vi "FPGAReadout.vi"() -> ()   [LabVIEW 2018]
uses:
  Downloads/hx711 myRIO/hx711/State.ctl
  Downloads/hx711 myRIO/hx711/Data.ctl
  <vilib>/rvi/Emulation/niFpgaGetClockAttributes.vi
  <vilib>/rvi/Emulation/niFpgaSctlEmulationGetInTimedLoop.vi
  <vilib>/rvi/Emulation/niFpgaEmulationReportErrorSimple.vi
  <vilib>/rvi/Emulation/niFpgaProcessEmulError.vi
  <vilib>/rvi/eio/common/nirviEmuTemplateMethod_errors.vi
  <vilib>/rvi/Emulation/niFpgaCriticalErrorInLSC.vi
  <vilib>/eio/EIONode/EIONode.xnode
panel:
  in  "PowerDown? 3":bool
  out "Data 3":i32
  in  "Gain/ChannelSelect 3":T1(ring)
  out "ConnectorA/DIO4":bool
  out "State 3":T2
  out "Data array3":i32[](array[numeric])
  in  "PowerDown? 2":bool
  out "Data 2":i32
  in  "Gain/ChannelSelect 2":T1(ring)
  out "ConnectorA/DIO2":bool
  out "State 2":T2
  out "Data array 2":i32[](array[numeric])
  out "RawCurrent":u16
  out "RawVoltage":i16
  out "State":T2
  out "ConnectorA/DIO0":bool
  out "Data array":i32[](array[numeric])
  in  "PowerDown?":bool
  out "Data":i32
  in  "Gain/ChannelSelect":T1(ring)
  in  "stop":bool
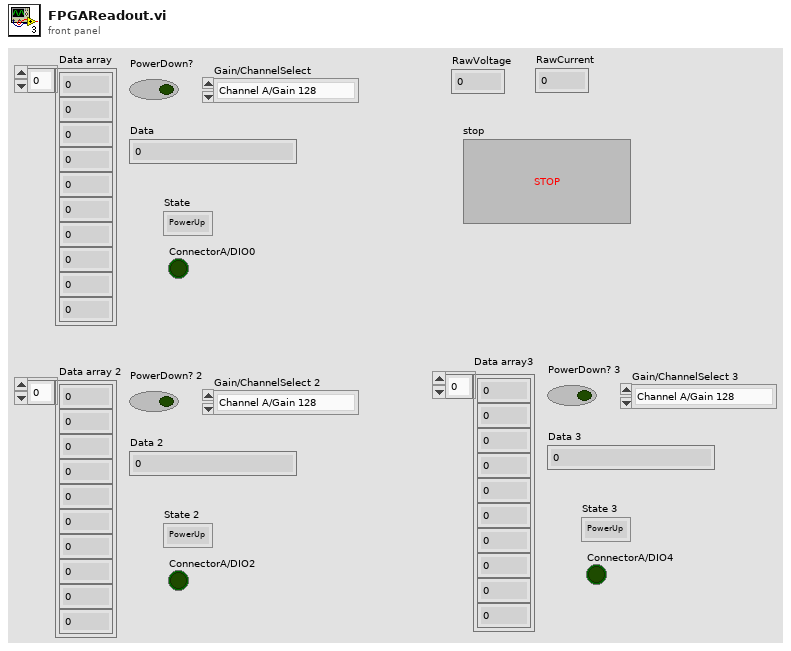
[diagram p1: front panel]
types:
  T1 = enum16{"Channel A/Gain 128", "Channel A/Gain 64", "Channel B/Gain 32"}
  T2 = typedef "State.ctl" = enum16{"PowerUp", "PowerDown", "Gain/ChannelSelect", "ReadData", "ClockLow", "ClockHigh", "ConvertData", "RetrievalReady?"}
  T3 = typedef "Data.ctl" = cluster{"DT":bool, "SCK":bool, "2's Data":i32, "PulseCount":u8, "DelayTime":u8, "Data":i32, "PowerDown?":bool, "Gain/ChannelSelect":enum16{"Channel A/Gain 128", "Channel A/Gain 64", "Channel B/Gain 32"}}
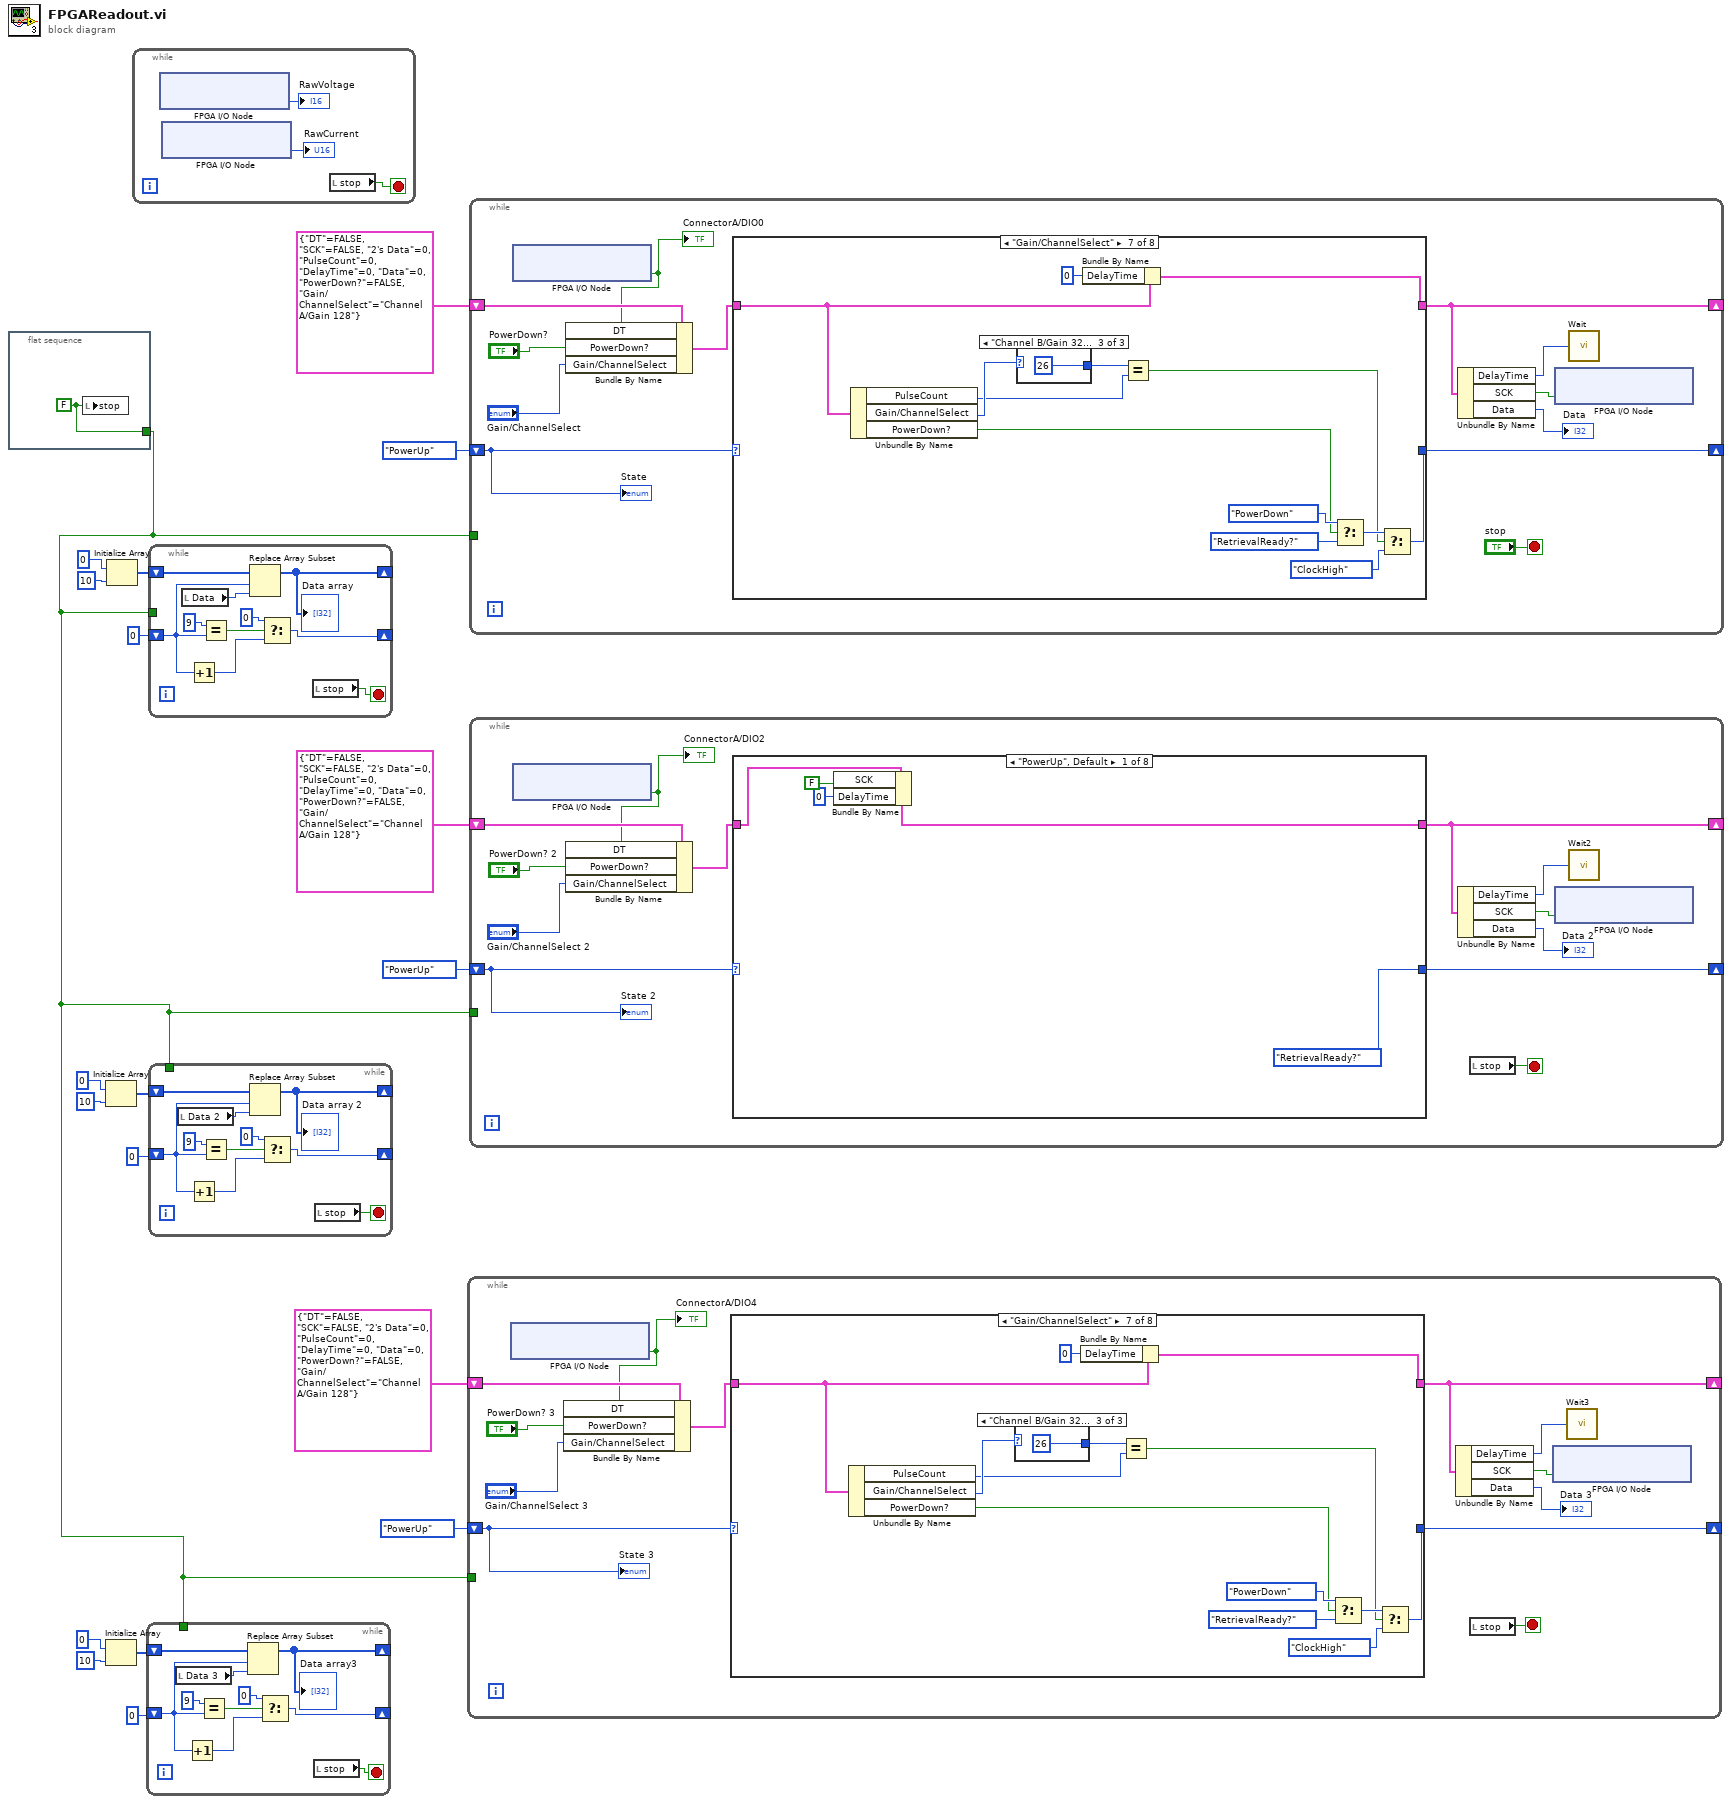
[diagram p0: block diagram]
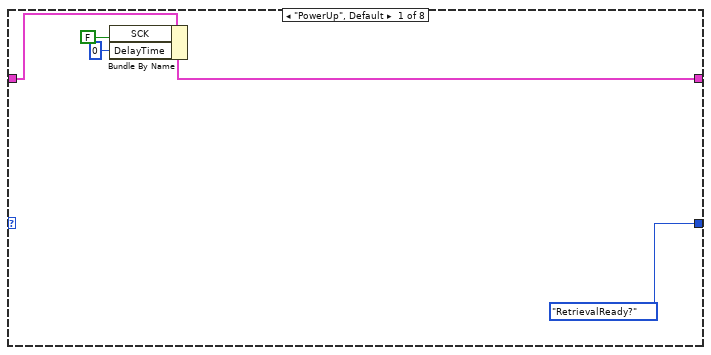
[diagram p2: hidden frame]
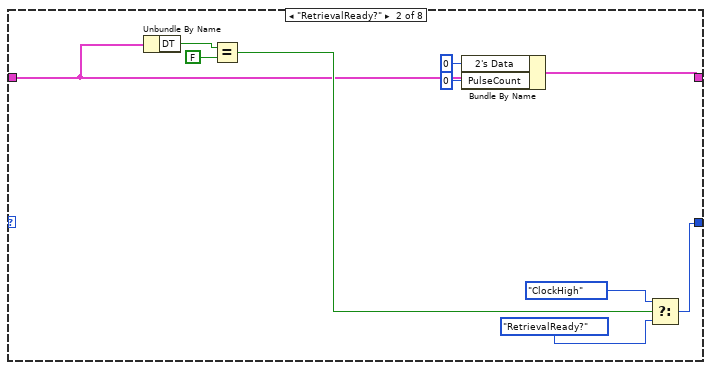
[diagram p3: hidden frame]
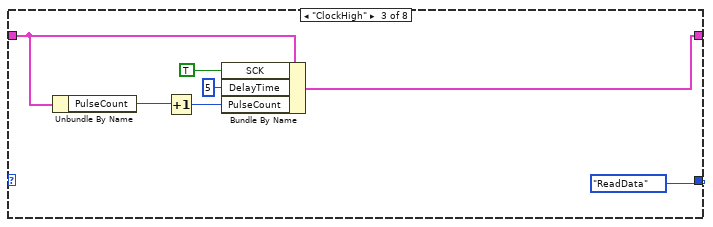
[diagram p4: hidden frame]
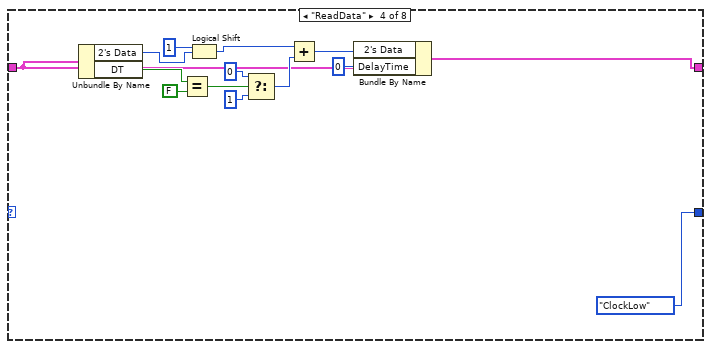
[diagram p5: hidden frame]
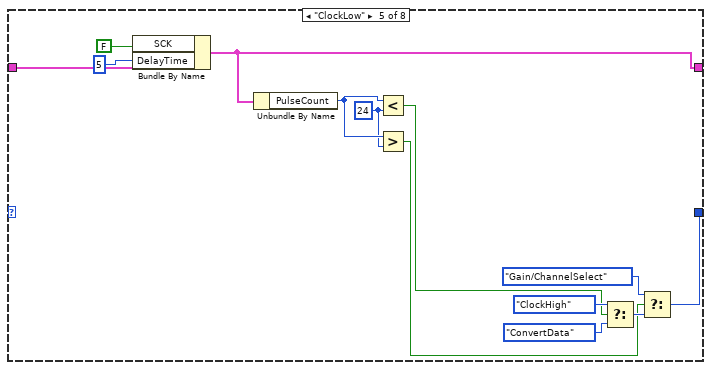
[diagram p6: hidden frame]
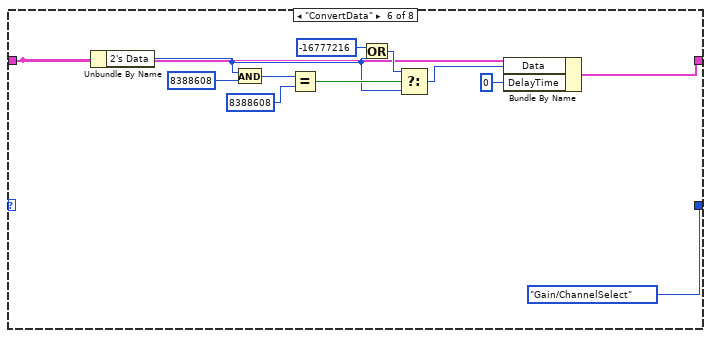
[diagram p7: hidden frame]
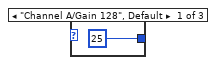
[diagram p8: hidden frame]
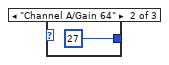
[diagram p9: hidden frame]
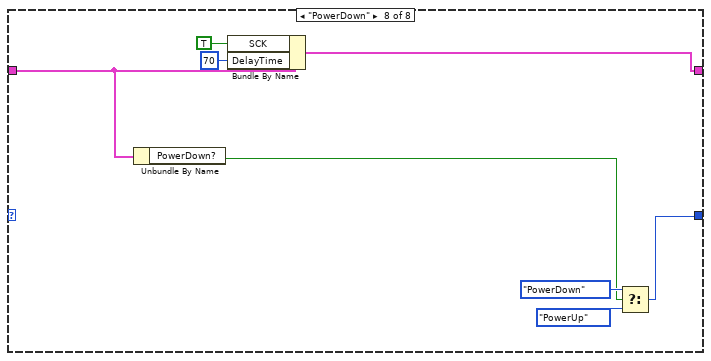
[diagram p10: hidden frame]
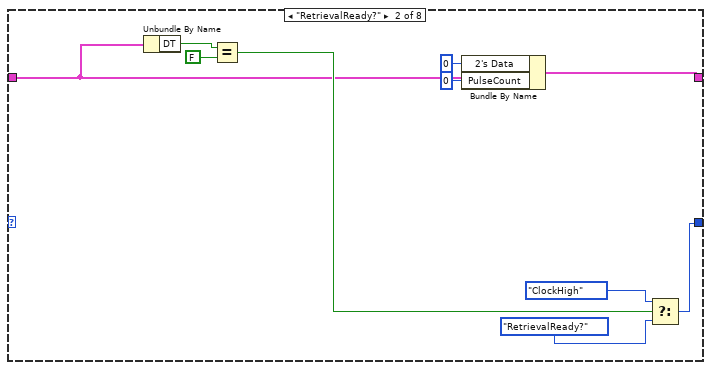
[diagram p11: hidden frame]
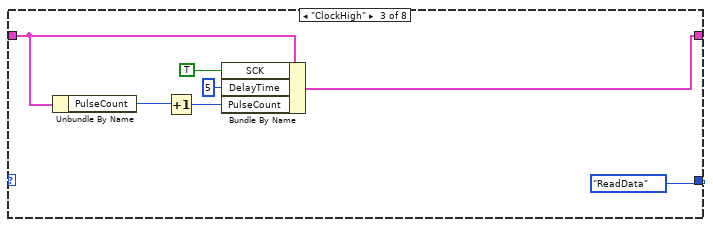
[diagram p12: hidden frame]
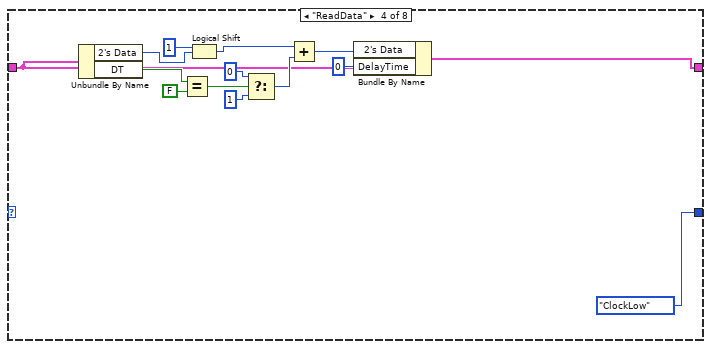
[diagram p13: hidden frame]
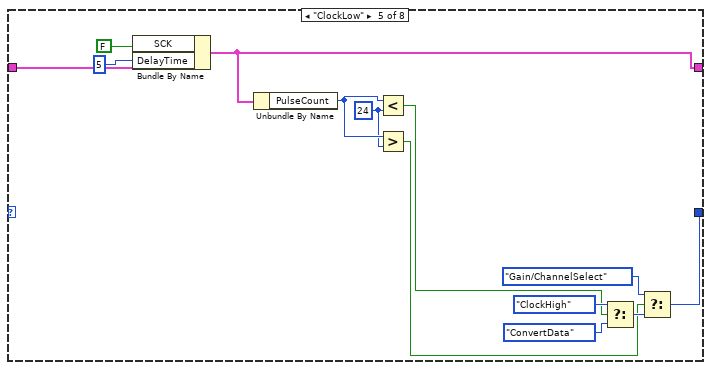
[diagram p14: hidden frame]
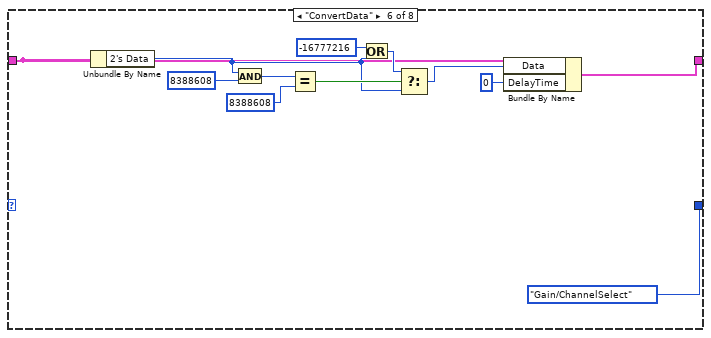
[diagram p15: hidden frame]
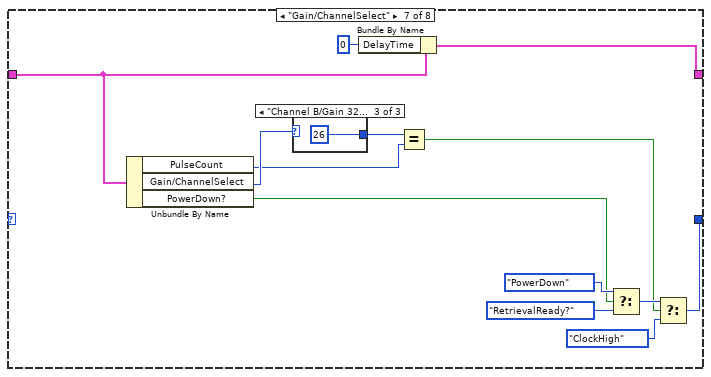
[diagram p16: hidden frame]
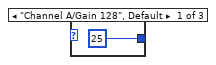
[diagram p17: hidden frame]
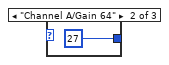
[diagram p18: hidden frame]
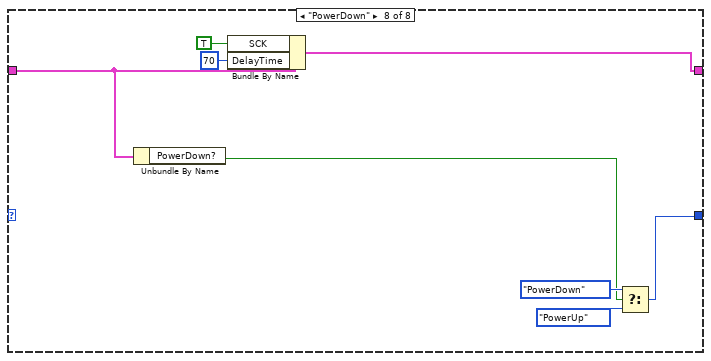
[diagram p19: hidden frame]
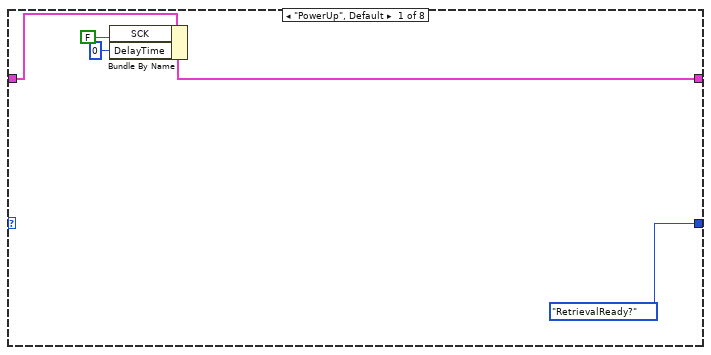
[diagram p20: hidden frame]
diagram:
  n1 = flat-sequence {
    tunnel: [w20] -> w9
    frame #0 {
      w20 = FALSE
      n2 = local write "stop"(w20) -> ()
    }
  }
  n3 = Initialize Array(0 ("Data"), 10 ("dimension size")) -> (w5:i32[])
  n4 = Initialize Array(0 ("Data"), 10 ("dimension size")) -> (w2:i32[])
  n5 = Initialize Array(0 ("Data"), 10 ("dimension size")) -> (w16:i32[])
  n6 = while {
    stop <- w21 stop-if-true
    n7 = xnode "FPGA I/O Node"() -> ("ConnectorC/AI0"=→"RawVoltage":i16)  [unwired: 1 in, 1 out]
    n8 = xnode "FPGA I/O Node"() -> ("ConnectorA/AI0"=→"RawCurrent":u16)  [unwired: 1 in, 1 out]
    n9 = local read "stop"() -> (w21:bool)
  }
  n10 = while {
    shift-right: [w25] -> _
    shift-left: w2 -> [w26]
    shift-right: [w31] -> _
    shift-left: 0 ("index") -> [w27]
    tunnel: w9 -> [_]
    stop <- w24 stop-if-true
    n11 = local read "Data 3"() -> (w33:i32)
    n12 = Increment(x=w27) -> (x+1=w30:i32)
    n13 = Equal?(x=9, y=w27) -> (x = y?=w28:bool)
    n14 = Replace Array Subset(array=w26, new element=w33, index=w27) -> (w25:i32[])
    "Data array3" <- w25
    n15 = Select(t=0 ("index"), s=w28, f=w30) -> (s? t:f=w31:i32)
    n16 = local read "stop"() -> (w24:bool)
  }
  n17 = while {
    shift-right: [w35] -> _
    shift-left: w16 -> [w36]
    shift-right: [w41] -> _
    shift-left: 0 ("index") -> [w37]
    tunnel: w9 -> [_]
    stop <- w34 stop-if-true
    n18 = local read "Data"() -> (w43:i32)
    n19 = Increment(x=w37) -> (x+1=w40:i32)
    n20 = Equal?(x=9, y=w37) -> (x = y?=w38:bool)
    n21 = Replace Array Subset(array=w36, new element=w43, index=w37) -> (w35:i32[])
    "Data array" <- w35
    n22 = Select(t=0 ("index"), s=w38, f=w40) -> (s? t:f=w41:i32)
    n23 = local read "stop"() -> (w34:bool)
  }
  n24 = while {
    shift-right: [w45] -> _
    shift-left: w5 -> [w46]
    shift-right: [w51] -> _
    shift-left: 0 ("index") -> [w47]
    tunnel: w9 -> [_]
    stop <- w44 stop-if-true
    n25 = local read "Data 2"() -> (w53:i32)
    n26 = Increment(x=w47) -> (x+1=w50:i32)
    n27 = Equal?(x=9, y=w47) -> (x = y?=w48:bool)
    n28 = Replace Array Subset(array=w46, new element=w53, index=w47) -> (w45:i32[])
    "Data array 2" <- w45
    n29 = Select(t=0 ("index"), s=w48, f=w50) -> (s? t:f=w51:i32)
    n30 = local read "stop"() -> (w44:bool)
  }
  n31 = while {
    shift-right: [w57] -> _
    shift-left: T3 {"DT"=FALSE, "SCK"=FALSE, "2's Data"=0, "PulseCount"=0, "DelayTime"=0, "Data"=0, "PowerDown?"=FALSE, "Gain/ChannelSelect"=enum."Channel A/Gain 128"} ("Data") -> [w62]
    shift-right: [w63] -> _
    shift-left: State."PowerUp" ("State") -> [w65]
    tunnel: w9 -> [_]
    stop <- w54 stop-if-true
    n32 = xnode "FPGA I/O Node"() -> ("ConnectorA/DIO4"=w60:bool)  [unwired: 1 in, 1 out]
    "ConnectorA/DIO4" <- w60
    n33 = Bundle By Name(cluster=w62, "DT"=w60, "PowerDown?"="PowerDown? 3", "Gain/ChannelSelect"="Gain/ChannelSelect 3") -> (w61:T3)
    n34 = case shown="\"Gain/ChannelSelect\"" w65 {
      tunnel: w61 -> [w70 w74 w83 w88 w114 w119 w129 w144]
      tunnel: [w68 w73 w87 w90 w109 w118 w128 w150] -> w57
      tunnel: [State."RetrievalReady?" ("State") w76 State."ReadData" ("State") State."ClockLow" ("State") w110 State."Gain/ChannelSelect" ("State") w136 w145] -> w63
      frame "PowerUp", Default {
        n35 = Bundle By Name(cluster=w70, "SCK"=FALSE, "DelayTime"=u8 0) -> (w68:T3)
      }
      frame "RetrievalReady?" {
        n36 = Unbundle By Name(w74) -> ("DT"=w80:bool)
        n37 = Equal?(x=w80, y=FALSE) -> (x = y?=w75:bool)
        n38 = Bundle By Name(cluster=w74, "2's Data"=0, "PulseCount"=u8 0) -> (w73:T3)
        n39 = Select(t=State."ClockHigh" ("State"), s=w75, f=State."RetrievalReady?" ("State")) -> (s? t:f=w76:T2)
      }
      frame "ClockHigh" {
        n40 = Unbundle By Name(w83) -> ("PulseCount"=w82:u8)
        n41 = Increment(x=w82) -> (x+1=w81:u8)
        n42 = Bundle By Name(cluster=w83, "SCK"=TRUE, "DelayTime"=u8 5, "PulseCount"=w81) -> (w87:T3)
      }
      frame "ReadData" {
        n43 = Unbundle By Name(w88) -> ("2's Data"=w101:i32, "DT"=w99:bool)
        n44 = Equal?(x=w99, y=FALSE ("SCK")) -> (x = y?=w97:bool)
        n45 = Logical Shift(y=i16 1, x=w101) -> (x << y=w96:i32)
        n46 = Select(t=0 ("DelayTime"), s=w97, f=1 ("DelayTime")) -> (s? t:f=w93:i32)
        n47 = Add(x=w96, y=w93) -> (x+y=w92:i32)
        n48 = Bundle By Name(cluster=w88, "2's Data"=w92, "DelayTime"=u8 0) -> (w90:T3)
      }
      frame "ClockLow" {
        w103 = u8 24 ("y")
        n49 = Bundle By Name(cluster=w114, "SCK"=FALSE, "DelayTime"=u8 5) -> (w109:T3)
        n50 = Unbundle By Name(w109) -> ("PulseCount"=w104:u8)
        n51 = Less?(x=w104, y=w103) -> (x < y?=w106:bool)
        n52 = Greater?(x=w104, y=w103) -> (0:w102:bool)
        n53 = Select(t=State."ClockHigh" ("State"), s=w106, f=State."ConvertData" ("State")) -> (s? t:f=w105:T2)
        n54 = Select(t=State."Gain/ChannelSelect" ("State"), s=w102, f=w105) -> (s? t:f=w110:T2)
      }
      frame "ConvertData" {
        n55 = Unbundle By Name(w119) -> ("2's Data"=w120:i32)
        n56 = And(x=w120, y=8388608) -> (x .and. y?=w125:i32)
        n57 = Equal?(x=w125, y=8388608) -> (x = y?=w123:bool)
        n58 = Or(x=-16777216 ("y"), y=w120) -> (x .or. y?=w121:i32)
        n59 = Select(t=w121, s=w123, f=w120) -> (s? t:f=w116:i32)
        n60 = Bundle By Name(cluster=w119, "Data"=w116, "DelayTime"=u8 0) -> (w118:T3)
      }
      frame "Gain/ChannelSelect" {
        n61 = Unbundle By Name(w129) -> ("PulseCount"=w132:u8, "Gain/ChannelSelect"=w134:T1, "PowerDown?"=w135:bool)
        n62 = case shown="\"Channel B/Gain 32\"" w134 {
          tunnel: [u8 25 ("PulseCount") u8 27 ("PulseCount") u8 26 ("PulseCount")] -> w133
          frame "Channel A/Gain 128", Default {
          }
          frame "Channel A/Gain 64" {
          }
          frame "Channel B/Gain 32" {
          }
        }
        n63 = Bundle By Name(cluster=w129, "DelayTime"=u8 0) -> (w128:T3)
        n64 = Equal?(x=w133, y=w132) -> (x = y?=w130:bool)
        n65 = Select(t=State."PowerDown" ("State"), s=w135, f=State."RetrievalReady?" ("State")) -> (s? t:f=w131:T2)
        n66 = Select(t=w131, s=w130, f=State."ClockHigh" ("State")) -> (s? t:f=w136:T2)
      }
      frame "PowerDown" {
        n67 = Unbundle By Name(w144) -> ("PowerDown?"=w143:bool)
        n68 = Bundle By Name(cluster=w144, "SCK"=TRUE, "DelayTime"=u8 70) -> (w150:T3)
        n69 = Select(t=State."PowerDown" ("State"), s=w143, f=State."PowerUp" ("State")) -> (s? t:f=w145:T2)
      }
    }
    n70 = Unbundle By Name(w57) -> ("DelayTime"=w64:u8, "SCK"=w56:bool, "Data"=→"Data 3":i32)
    n71 = local read "stop"() -> (w54:bool)
    n72 = xnode "FPGA I/O Node"("ConnectorA/DIO5"=w56) -> ()  [unwired: 1 in, 1 out]
    n73 = call "Wait3"("Count(uSec)"=w64) -> ()  [unwired: 1 out]
    "State 3" <- w65
  }
  n74 = while {
    shift-right: [w153] -> _
    shift-left: T3 {"DT"=FALSE, "SCK"=FALSE, "2's Data"=0, "PulseCount"=0, "DelayTime"=0, "Data"=0, "PowerDown?"=FALSE, "Gain/ChannelSelect"=enum."Channel A/Gain 128"} ("Data") -> [w159]
    shift-right: [w160] -> _
    shift-left: State."PowerUp" ("State") -> [w162]
    tunnel: w9 -> [_]
    stop <- "stop" stop-if-true
    n75 = xnode "FPGA I/O Node"() -> ("ConnectorA/DIO0"=w157:bool)  [unwired: 1 in, 1 out]
    "ConnectorA/DIO0" <- w157
    n76 = Bundle By Name(cluster=w159, "DT"=w157, "PowerDown?"="PowerDown?", "Gain/ChannelSelect"="Gain/ChannelSelect") -> (w158:T3)
    n77 = case shown="\"Gain/ChannelSelect\"" w162 {
      tunnel: w158 -> [w167 w171 w180 w185 w211 w216 w226 w241]
      tunnel: [w165 w170 w184 w187 w206 w215 w225 w247] -> w153
      tunnel: [State."RetrievalReady?" ("State") w173 State."ReadData" ("State") State."ClockLow" ("State") w207 State."Gain/ChannelSelect" ("State") w233 w242] -> w160
      frame "PowerUp", Default {
        n78 = Bundle By Name(cluster=w167, "SCK"=FALSE, "DelayTime"=u8 0) -> (w165:T3)
      }
      frame "RetrievalReady?" {
        n79 = Unbundle By Name(w171) -> ("DT"=w177:bool)
        n80 = Equal?(x=w177, y=FALSE) -> (x = y?=w172:bool)
        n81 = Bundle By Name(cluster=w171, "2's Data"=0, "PulseCount"=u8 0) -> (w170:T3)
        n82 = Select(t=State."ClockHigh" ("State"), s=w172, f=State."RetrievalReady?" ("State")) -> (s? t:f=w173:T2)
      }
      frame "ClockHigh" {
        n83 = Unbundle By Name(w180) -> ("PulseCount"=w179:u8)
        n84 = Increment(x=w179) -> (x+1=w178:u8)
        n85 = Bundle By Name(cluster=w180, "SCK"=TRUE, "DelayTime"=u8 5, "PulseCount"=w178) -> (w184:T3)
      }
      frame "ReadData" {
        n86 = Unbundle By Name(w185) -> ("2's Data"=w198:i32, "DT"=w196:bool)
        n87 = Equal?(x=w196, y=FALSE ("SCK")) -> (x = y?=w194:bool)
        n88 = Logical Shift(y=i16 1, x=w198) -> (x << y=w193:i32)
        n89 = Select(t=0 ("DelayTime"), s=w194, f=1 ("DelayTime")) -> (s? t:f=w190:i32)
        n90 = Add(x=w193, y=w190) -> (x+y=w189:i32)
        n91 = Bundle By Name(cluster=w185, "2's Data"=w189, "DelayTime"=u8 0) -> (w187:T3)
      }
      frame "ClockLow" {
        w200 = u8 24 ("y")
        n92 = Bundle By Name(cluster=w211, "SCK"=FALSE, "DelayTime"=u8 5) -> (w206:T3)
        n93 = Unbundle By Name(w206) -> ("PulseCount"=w201:u8)
        n94 = Less?(x=w201, y=w200) -> (x < y?=w203:bool)
        n95 = Greater?(x=w201, y=w200) -> (0:w199:bool)
        n96 = Select(t=State."ClockHigh" ("State"), s=w203, f=State."ConvertData" ("State")) -> (s? t:f=w202:T2)
        n97 = Select(t=State."Gain/ChannelSelect" ("State"), s=w199, f=w202) -> (s? t:f=w207:T2)
      }
      frame "ConvertData" {
        n98 = Unbundle By Name(w216) -> ("2's Data"=w217:i32)
        n99 = And(x=w217, y=8388608) -> (x .and. y?=w222:i32)
        n100 = Equal?(x=w222, y=8388608) -> (x = y?=w220:bool)
        n101 = Or(x=-16777216 ("y"), y=w217) -> (x .or. y?=w218:i32)
        n102 = Select(t=w218, s=w220, f=w217) -> (s? t:f=w213:i32)
        n103 = Bundle By Name(cluster=w216, "Data"=w213, "DelayTime"=u8 0) -> (w215:T3)
      }
      frame "Gain/ChannelSelect" {
        n104 = Unbundle By Name(w226) -> ("PulseCount"=w229:u8, "Gain/ChannelSelect"=w231:T1, "PowerDown?"=w232:bool)
        n105 = case shown="\"Channel B/Gain 32\"" w231 {
          tunnel: [u8 25 ("PulseCount") u8 27 ("PulseCount") u8 26 ("PulseCount")] -> w230
          frame "Channel A/Gain 128", Default {
          }
          frame "Channel A/Gain 64" {
          }
          frame "Channel B/Gain 32" {
          }
        }
        n106 = Bundle By Name(cluster=w226, "DelayTime"=u8 0) -> (w225:T3)
        n107 = Equal?(x=w230, y=w229) -> (x = y?=w227:bool)
        n108 = Select(t=State."PowerDown" ("State"), s=w232, f=State."RetrievalReady?" ("State")) -> (s? t:f=w228:T2)
        n109 = Select(t=w228, s=w227, f=State."ClockHigh" ("State")) -> (s? t:f=w233:T2)
      }
      frame "PowerDown" {
        n110 = Unbundle By Name(w241) -> ("PowerDown?"=w240:bool)
        n111 = Bundle By Name(cluster=w241, "SCK"=TRUE, "DelayTime"=u8 70) -> (w247:T3)
        n112 = Select(t=State."PowerDown" ("State"), s=w240, f=State."PowerUp" ("State")) -> (s? t:f=w242:T2)
      }
    }
    n113 = Unbundle By Name(w153) -> ("DelayTime"=w161:u8, "SCK"=w152:bool, "Data"=→"Data":i32)
    n114 = xnode "FPGA I/O Node"("ConnectorA/DIO1"=w152) -> ()  [unwired: 1 in, 1 out]
    n115 = call "Wait"("Count(uSec)"=w161) -> ()  [unwired: 1 out]
    "State" <- w162
  }
  n116 = while {
    shift-right: [w251] -> _
    shift-left: T3 {"DT"=FALSE, "SCK"=FALSE, "2's Data"=0, "PulseCount"=0, "DelayTime"=0, "Data"=0, "PowerDown?"=FALSE, "Gain/ChannelSelect"=enum."Channel A/Gain 128"} ("Data") -> [w256]
    shift-right: [w257] -> _
    shift-left: State."PowerUp" ("State") -> [w259]
    tunnel: w9 -> [_]
    stop <- w248 stop-if-true
    n117 = xnode "FPGA I/O Node"() -> ("ConnectorA/DIO2"=w254:bool)  [unwired: 1 in, 1 out]
    "ConnectorA/DIO2" <- w254
    n118 = Bundle By Name(cluster=w256, "DT"=w254, "PowerDown?"="PowerDown? 2", "Gain/ChannelSelect"="Gain/ChannelSelect 2") -> (w255:T3)
    n119 = case shown="\"PowerUp\", Default" w259 {
      tunnel: w255 -> [w264 w268 w277 w282 w308 w313 w323 w338]
      tunnel: [w262 w267 w281 w284 w303 w312 w322 w344] -> w251
      tunnel: [State."RetrievalReady?" ("State") w270 State."ReadData" ("State") State."ClockLow" ("State") w304 State."Gain/ChannelSelect" ("State") w330 w339] -> w257
      frame "PowerUp", Default {
        n120 = Bundle By Name(cluster=w264, "SCK"=FALSE, "DelayTime"=u8 0) -> (w262:T3)
      }
      frame "RetrievalReady?" {
        n121 = Unbundle By Name(w268) -> ("DT"=w274:bool)
        n122 = Equal?(x=w274, y=FALSE) -> (x = y?=w269:bool)
        n123 = Bundle By Name(cluster=w268, "2's Data"=0, "PulseCount"=u8 0) -> (w267:T3)
        n124 = Select(t=State."ClockHigh" ("State"), s=w269, f=State."RetrievalReady?" ("State")) -> (s? t:f=w270:T2)
      }
      frame "ClockHigh" {
        n125 = Unbundle By Name(w277) -> ("PulseCount"=w276:u8)
        n126 = Increment(x=w276) -> (x+1=w275:u8)
        n127 = Bundle By Name(cluster=w277, "SCK"=TRUE, "DelayTime"=u8 5, "PulseCount"=w275) -> (w281:T3)
      }
      frame "ReadData" {
        n128 = Unbundle By Name(w282) -> ("2's Data"=w295:i32, "DT"=w293:bool)
        n129 = Equal?(x=w293, y=FALSE ("SCK")) -> (x = y?=w291:bool)
        n130 = Logical Shift(y=i16 1, x=w295) -> (x << y=w290:i32)
        n131 = Select(t=0 ("DelayTime"), s=w291, f=1 ("DelayTime")) -> (s? t:f=w287:i32)
        n132 = Add(x=w290, y=w287) -> (x+y=w286:i32)
        n133 = Bundle By Name(cluster=w282, "2's Data"=w286, "DelayTime"=u8 0) -> (w284:T3)
      }
      frame "ClockLow" {
        w297 = u8 24 ("y")
        n134 = Bundle By Name(cluster=w308, "SCK"=FALSE, "DelayTime"=u8 5) -> (w303:T3)
        n135 = Unbundle By Name(w303) -> ("PulseCount"=w298:u8)
        n136 = Less?(x=w298, y=w297) -> (x < y?=w300:bool)
        n137 = Greater?(x=w298, y=w297) -> (0:w296:bool)
        n138 = Select(t=State."ClockHigh" ("State"), s=w300, f=State."ConvertData" ("State")) -> (s? t:f=w299:T2)
        n139 = Select(t=State."Gain/ChannelSelect" ("State"), s=w296, f=w299) -> (s? t:f=w304:T2)
      }
      frame "ConvertData" {
        n140 = Unbundle By Name(w313) -> ("2's Data"=w314:i32)
        n141 = And(x=w314, y=8388608) -> (x .and. y?=w319:i32)
        n142 = Equal?(x=w319, y=8388608) -> (x = y?=w317:bool)
        n143 = Or(x=-16777216 ("y"), y=w314) -> (x .or. y?=w315:i32)
        n144 = Select(t=w315, s=w317, f=w314) -> (s? t:f=w310:i32)
        n145 = Bundle By Name(cluster=w313, "Data"=w310, "DelayTime"=u8 0) -> (w312:T3)
      }
      frame "Gain/ChannelSelect" {
        n146 = Unbundle By Name(w323) -> ("PulseCount"=w326:u8, "Gain/ChannelSelect"=w328:T1, "PowerDown?"=w329:bool)
        n147 = case shown="\"Channel B/Gain 32\"" w328 {
          tunnel: [u8 25 ("PulseCount") u8 27 ("PulseCount") u8 26 ("PulseCount")] -> w327
          frame "Channel A/Gain 128", Default {
          }
          frame "Channel A/Gain 64" {
          }
          frame "Channel B/Gain 32" {
          }
        }
        n148 = Bundle By Name(cluster=w323, "DelayTime"=u8 0) -> (w322:T3)
        n149 = Equal?(x=w327, y=w326) -> (x = y?=w324:bool)
        n150 = Select(t=State."PowerDown" ("State"), s=w329, f=State."RetrievalReady?" ("State")) -> (s? t:f=w325:T2)
        n151 = Select(t=w325, s=w324, f=State."ClockHigh" ("State")) -> (s? t:f=w330:T2)
      }
      frame "PowerDown" {
        n152 = Unbundle By Name(w338) -> ("PowerDown?"=w337:bool)
        n153 = Bundle By Name(cluster=w338, "SCK"=TRUE, "DelayTime"=u8 70) -> (w344:T3)
        n154 = Select(t=State."PowerDown" ("State"), s=w337, f=State."PowerUp" ("State")) -> (s? t:f=w339:T2)
      }
    }
    n155 = Unbundle By Name(w251) -> ("DelayTime"=w258:u8, "SCK"=w250:bool, "Data"=→"Data 2":i32)
    n156 = local read "stop"() -> (w248:bool)
    n157 = xnode "FPGA I/O Node"("ConnectorA/DIO3"=w250) -> ()  [unwired: 1 in, 1 out]
    n158 = call "Wait2"("Count(uSec)"=w258) -> ()  [unwired: 1 out]
    "State 2" <- w259
  }
